vi "OpenConnection.vi"(8 "error in (no error)":errorcluster, 9 "Timeout (ms)":u32=5000 min=1, 10 "Connection Params":T1={"Vid"=0, "Pid"=0, "Device Index"=0, "u32_I2Cclk"=100} {"u32_I2Cclk" min=100 max=4000 step=1 format="%d Kbps"; "Pid" format="%.0x"; "Vid" format="%.0x"}, 11 "II2COUSB in":refnum<class "II2COUSB.lvclass">) -> (0 "error out":errorcluster, 3 "II2COUSB out":refnum<class "II2COUSB.lvclass">)   [LabVIEW 2020, in "II2COUSB.lvlib" / "II2COUSB.lvclass"]
doc: "Open connection"
uses:
  II2COUSB.lvclass
  ConnectionParams.ctl
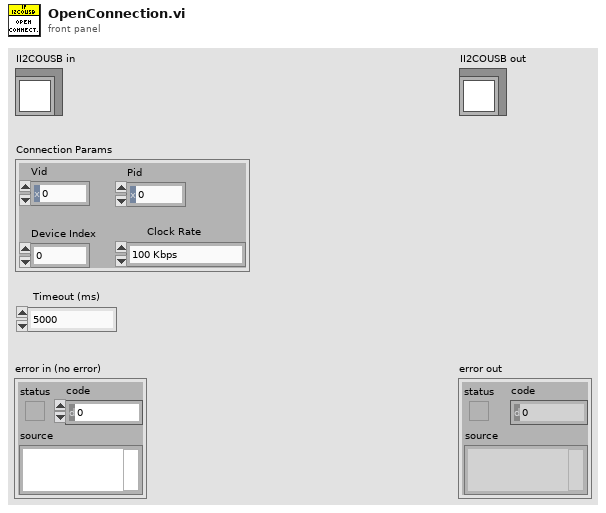
[diagram p1: front panel]
types:
  T1 = typedef "II2COUSB.lvlib/II2COUSB.lvclass/ConnectionParams.ctl" = cluster{"Vid":u16, "Pid":u16, "Device Index":u32, "u32_I2Cclk":u32}
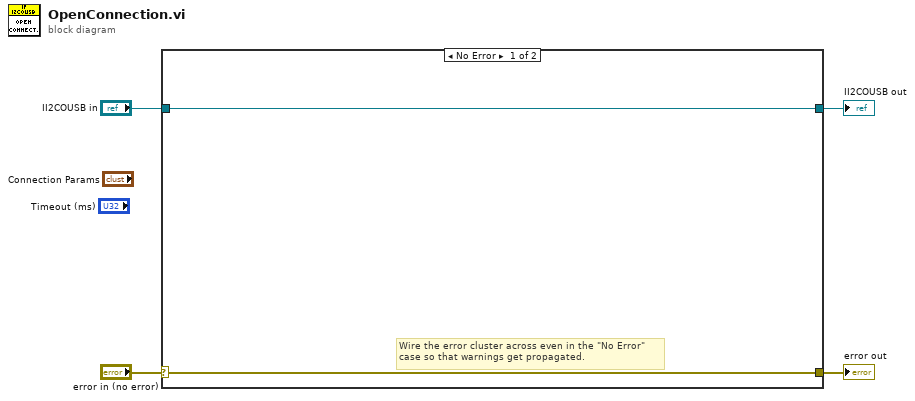
[diagram p0: block diagram]
diagram:
  n1 = case shown="No Error" "error in (no error)" {
    selector: "error in (no error)" -> [w5 w8]
    tunnel: [w5 w8] -> w3
    tunnel: [w6 w7] -> w1
    tunnel: "II2COUSB in" -> [w6 w7]
    frame No Error {
      # "Wire the error cluster across even in the \"No Error\"\ncase so that warnings get propagated."
    }
    frame Error {
    }
  }
  "error out" <- w3
  "II2COUSB out" <- w1
